vi "GET.vi"(6 "timeout (10000)":i32=10000, 7 "output file":path=path "", 8 "error in (no error)":errorcluster, 10 "url":string, 11 "HTTP Client reqwest in":refnum<class "HTTP Client reqwest.lvclass">) -> (0 "error out":errorcluster, 1 "body":string, 2 "headers":string, 3 "HTTP Client reqwest out":refnum<class "HTTP Client reqwest.lvclass">)   [LabVIEW 2021, in "HTTP Client reqwest.lvclass"]
uses:
  HTTP Client reqwest.lvclass
  HTTP Client reqwest.lvclass/HTTP Client reqwest.ctl
  external/reqwest-rs-labview/lv_src/Types/http_method_enum.ctl
  external/reqwest-rs-labview/lv_src/RequestBuilder/RequestBuilder.lvclass
  external/reqwest-rs-labview/lv_src/Client/Client.lvclass
  external/reqwest-rs-labview/lv_src/reqwest.lvlib
  external/reqwest-rs-labview/lv_src/Request/Request.lvclass
  external/reqwest-rs-labview/lv_src/Headers/Headers.lvclass
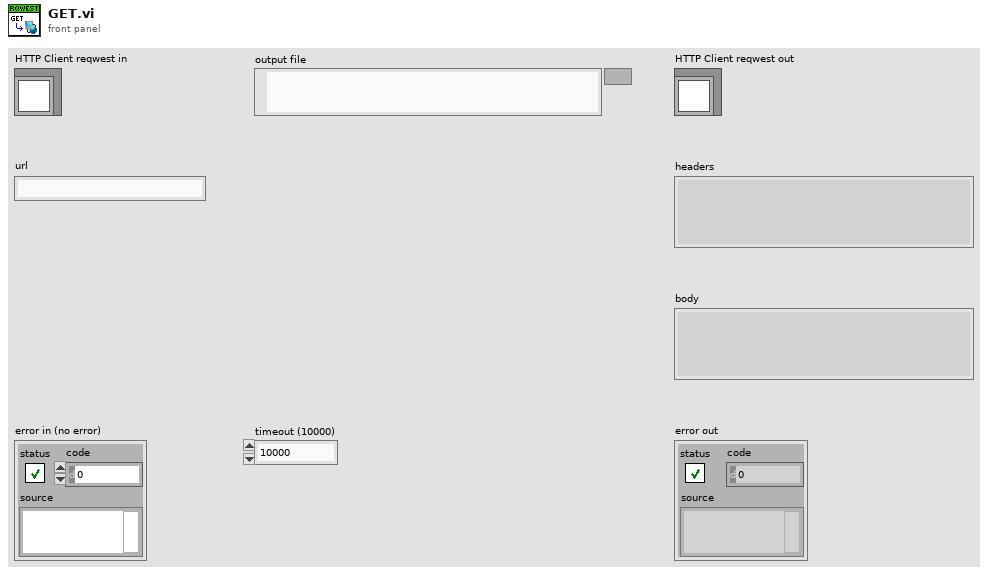
[diagram p1: front panel]
types:
  T1 = typedef "reqwest.lvlib/http_method_enum.ctl" = enum8{"<select>", "GET", "POST", "PUT", "DELETE", "HEAD", "OPTIONS", "CONNECT", "PATCH", "TRACE"}
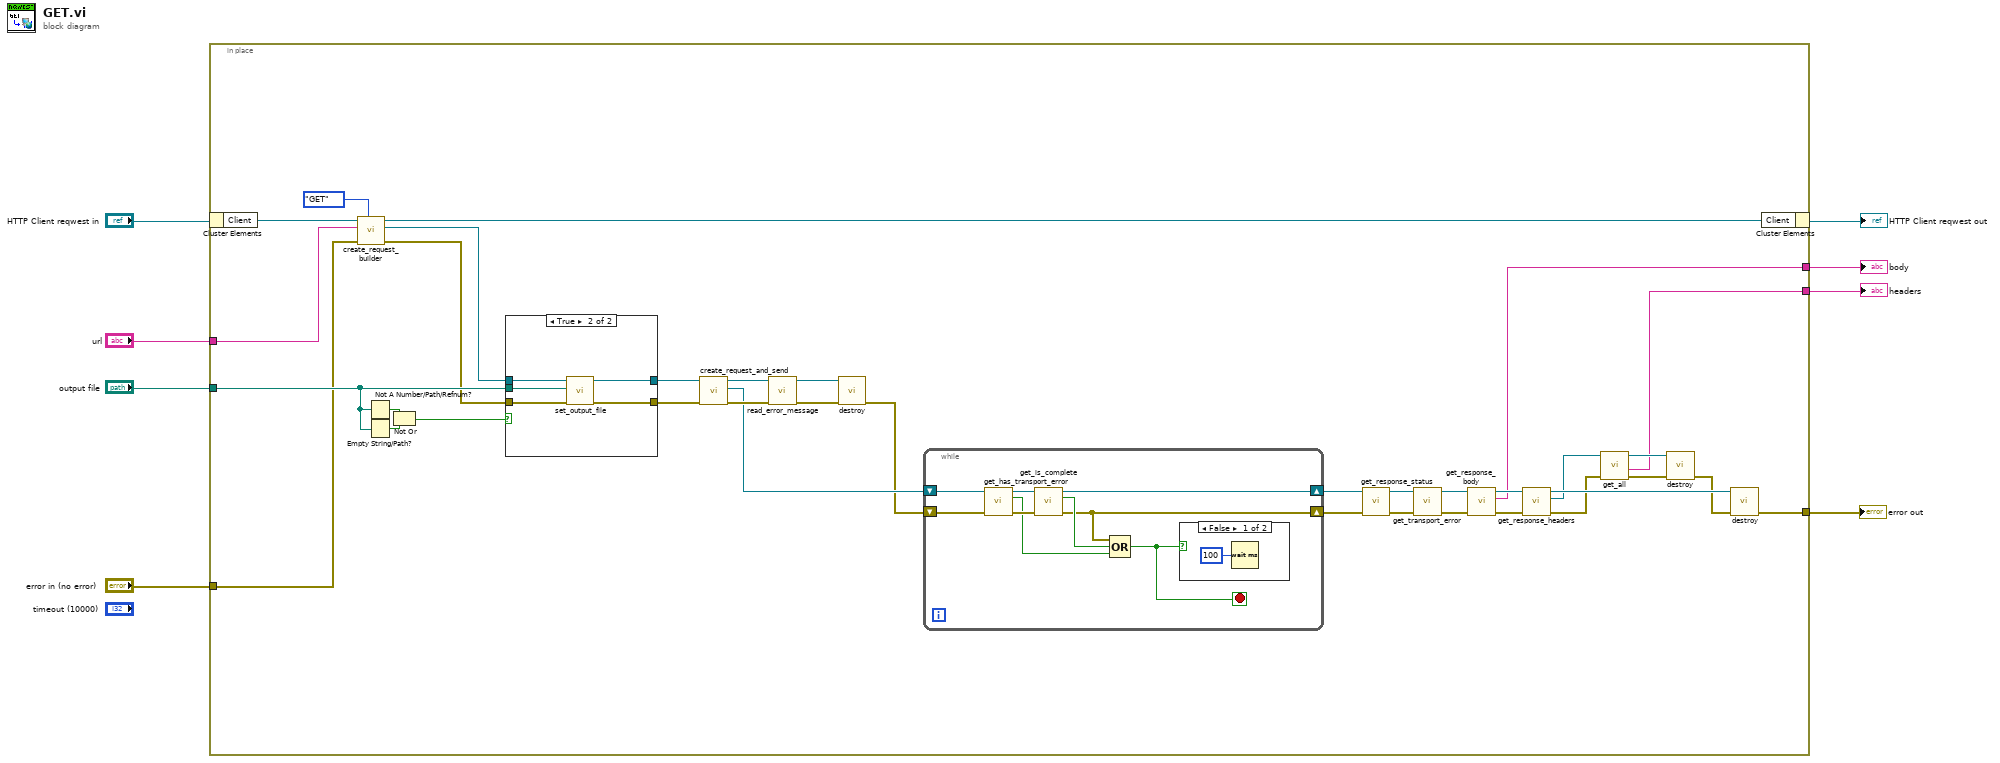
[diagram p0: block diagram]
diagram:
  n1 = in-place {
    in-place-border: "url" -> [w42]
    in-place-border: "output file" -> [w37]
    in-place-border: "error in (no error)" -> [w36]
    in-place-border: [w12] -> w3
    in-place-border: [w10] -> w2
    in-place-border: [w9] -> w1
    n2 = in-place-cluster #1("HTTP Client reqwest in") -> ("Client"=w43:refnum<class "Client.lvclass">)
    n3 = call "create_request_builder.vi"("HTTP Method"=http_method_enum."GET", "error in (no error)"=w36, "url"=w42, "Client in"=w43) -> ("error out"=w35:errorcluster, "RequestBuilder out"=w38:refnum<class "RequestBuilder.lvclass">, "Client out"=w11:refnum<class "Client.lvclass">)  [unwired: 5 in]
    n4 = Not A Number/Path/Refnum?(number/path/refnum=w37) -> (NaN/Path/Refnum?=w40:bool)
    n5 = Empty String/Path?(string/path=w37) -> (empty?=w41:bool)
    n6 = Not Or(1:w41, 2:w40) -> (0:w39:bool)
    n7 = case shown="True" w39 {
      tunnel: w38 -> [w45 w51]
      tunnel: w37 -> [_ w50]
      tunnel: [w45 w49] -> w34
      tunnel: w35 -> [w46 w48]
      tunnel: [w46 w47] -> w33
      frame False {
      }
      frame True {
        n8 = call "set_output_file.vi"("error in (no error)"=w48, "output_file"=w50, "obj in"=w51) -> ("error out"=w47:errorcluster, "obj out"=w49:refnum<class "RequestBuilder.lvclass">)  [unwired: 6 in, 1 out]
      }
    }
    n9 = call "create_request_and_send.vi"("error in"=w33, "obj in"=w34) -> ("error out"=w32:errorcluster, "request"=w28:refnum<class "Request.lvclass">, "obj out"=w31:refnum<class "RequestBuilder.lvclass">)  [unwired: 7 in]
    n10 = call "read_error_message.vi"("error in (no error)"=w32, "RequestBuilder in"=w31) -> ("error out"=w30:errorcluster, "RequestBuilder in"=w29:refnum<class "RequestBuilder.lvclass">)  [unwired: 7 in, 1 out]
    n11 = call "destroy.vi"("error in"=w30, "RequestBuilder in"=w29) -> ("error out"=w27:errorcluster)  [unwired: 8 in, 1 out]
    n12 = while {
      shift-right: [w54] -> w13
      shift-left: w28 -> [w59]
      shift-right: [w53] -> w14
      shift-left: w27 -> [w58]
      stop <- w52 stop-if-true
      n13 = call "get_has_transport_error.vi"("error in (no error)"=w58, "Request in"=w59) -> ("error out"=w56:errorcluster, "has_transport_error"=w55:bool, "Request out"=w57:refnum<class "Request.lvclass">)  [unwired: 7 in]
      n14 = call "get_is_complete.vi"("error in (no error)"=w56, "Request in"=w57) -> ("error out"=w53:errorcluster, "is_complete"=w60:bool, "Request out"=w54:refnum<class "Request.lvclass">)  [unwired: 7 in]
      n15 = Compound Arithmetic op=OR(w53, w60, w55) -> (w52:bool)
      n16 = case shown="False" w52 {
        frame False {
          n17 = Wait (ms)(milliseconds to wait=u32 100) -> ()  [unwired: 1 out]
        }
        frame True {
        }
      }
    }
    n18 = call "get_response_status.vi"("error in (no error)"=w14, "Request in"=w13) -> ("error out"=w16:errorcluster, "Request out"=w15:refnum<class "Request.lvclass">)  [unwired: 7 in, 1 out]
    n19 = call "get_transport_error.vi"("error in (no error)"=w16, "Request in"=w15) -> ("error out"=w17:errorcluster, "Request in"=w18:refnum<class "Request.lvclass">)  [unwired: 7 in, 1 out]
    n20 = call "get_response_body.vi"("error in (no error)"=w17, "Request in"=w18) -> ("error out"=w24:errorcluster, "string_value"=w10:string, "Request in"=w26:refnum<class "Request.lvclass">)  [unwired: 7 in]
    n21 = call "get_response_headers.vi"("error in (no error)"=w24, "Request in"=w26) -> ("error out"=w22:errorcluster, "response_headers"=w23:refnum<class "Headers.lvclass">, "Request in"=w25:refnum<class "Request.lvclass">)  [unwired: 7 in]
    n22 = call "get_all.vi"("error in (no error)"=w22, "Headers in"=w23) -> ("error out"=w20:errorcluster, "headers"=w9:string, "Headers in"=w21:refnum<class "Headers.lvclass">)  [unwired: 6 in, 1 out]
    n23 = call "destroy.vi"("error in (no error)"=w20, "Headers in"=w21) -> ("error out"=w19:errorcluster)  [unwired: 9 in]
    n24 = call "destroy.vi"("error in (no error)"=w19, "Request in"=w25) -> ("error out"=w12:errorcluster)  [unwired: 8 in, 1 out]
    n25 = in-place-cluster #1("Client"=w11) -> (→"HTTP Client reqwest out":refnum<class "HTTP Client reqwest.lvclass">)
  }
  "error out" <- w3
  "headers" <- w1
  "body" <- w2
